vi "nonZeroInc.vi"(1 "inc.":dbl) -> (0 "non-zero inc.":dbl)   [LabVIEW 2015]
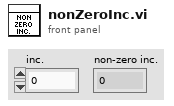
[diagram p1: front panel]
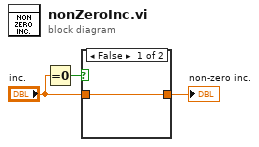
[diagram p0: block diagram]
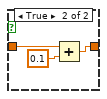
[diagram p2: hidden frame]
diagram:
  n1 = Equal To 0?(x="inc.") -> (x = 0?=w3:bool)
  n2 = case shown="False" w3 {
    tunnel: "inc." -> [w4 w7]
    tunnel: [w4 w5] -> w1
    frame False {
    }
    frame True {
      n3 = Add(x=w7, y=0.1) -> (x+y=w5:dbl)
    }
  }
  "non-zero inc." <- w1
